vi "General - String to Boolean.vi"(4 "Text In":string) -> (1 "Boolean Out":bool)   [LabVIEW 2018]
doc: "Converts a string to a boolean. The output is TRUE if the string input is \"TRUE\", \"T\", \"1\", \"PASS\" or \"P\"."
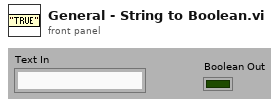
[diagram p1: front panel]
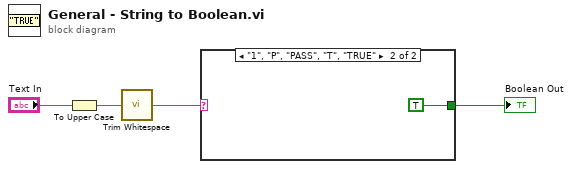
[diagram p0: block diagram]
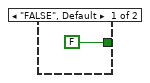
[diagram p2: hidden frame]
diagram:
  n1 = To Upper Case(1:"Text In") -> (0:w3:string)
  n2 = call <vilib>:"Trim Whitespace.vi"("string"=w3) -> ("trimmed string"=w2:string)  [unwired: 1 in]
  n3 = case shown="\"1\", \"P\", \"PASS\", \"T\", \"TRUE\"" w2 {
    tunnel: [FALSE TRUE] -> w1
    frame "FALSE", Default {
    }
    frame "1", "P", "PASS", "T", "TRUE" {
    }
  }
  "Boolean Out" <- w1
